vi "Write I16.vi"(6 "wait for reply (T)":bool=TRUE, 7 "Data":i16, 8 "error in":errorcluster, 9 "Variable":string, 10 "Drive":string) -> (0 "error out":errorcluster, 1 "timed out?":bool)   [LabVIEW 2024, in "Hardware Controller.lvlib"]
doc: "This event will pass on the data to be written to the ethercat module\n_____\nCreated using DQMH Event Scripter 7.0.0.1280."
uses:
  Hardware Controller.lvlib
  Write I16 Argument--cluster.ctl
  Write I16 (Reply Payload)--cluster.ctl
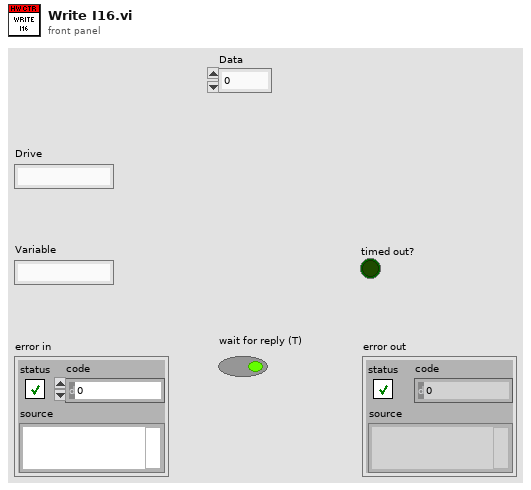
[diagram p1: front panel]
types:
  T1 = typedef "Hardware Controller.lvlib/Write I16 Argument--cluster.ctl" = cluster{"Drive":string, "Variable":string, "Data":i16, "Wait Notifier":refnum<notifier>, "wait for reply":bool}
  T2 = typedef "Hardware Controller.lvlib/Request Events--cluster.ctl" = cluster{"Stop Module":refnum<user-event>, "Show Panel":refnum<user-event>, "Hide Panel":refnum<user-event>, "Get Module Execution Status":refnum<user-event>, "Show Diagram":refnum<user-event>, "Private":cluster{"Start System State Broadcast Helper Loop":refnum<user-event>, "Launch EtherCat":refnum<user-event>}, "Launch all Hardware":refnum<user-event>, "Write I16":refnum<user-event>}
  T3 = typedef "Hardware Controller.lvlib/Write I16 (Reply Payload)--cluster.ctl" = cluster{"error":errorcluster}
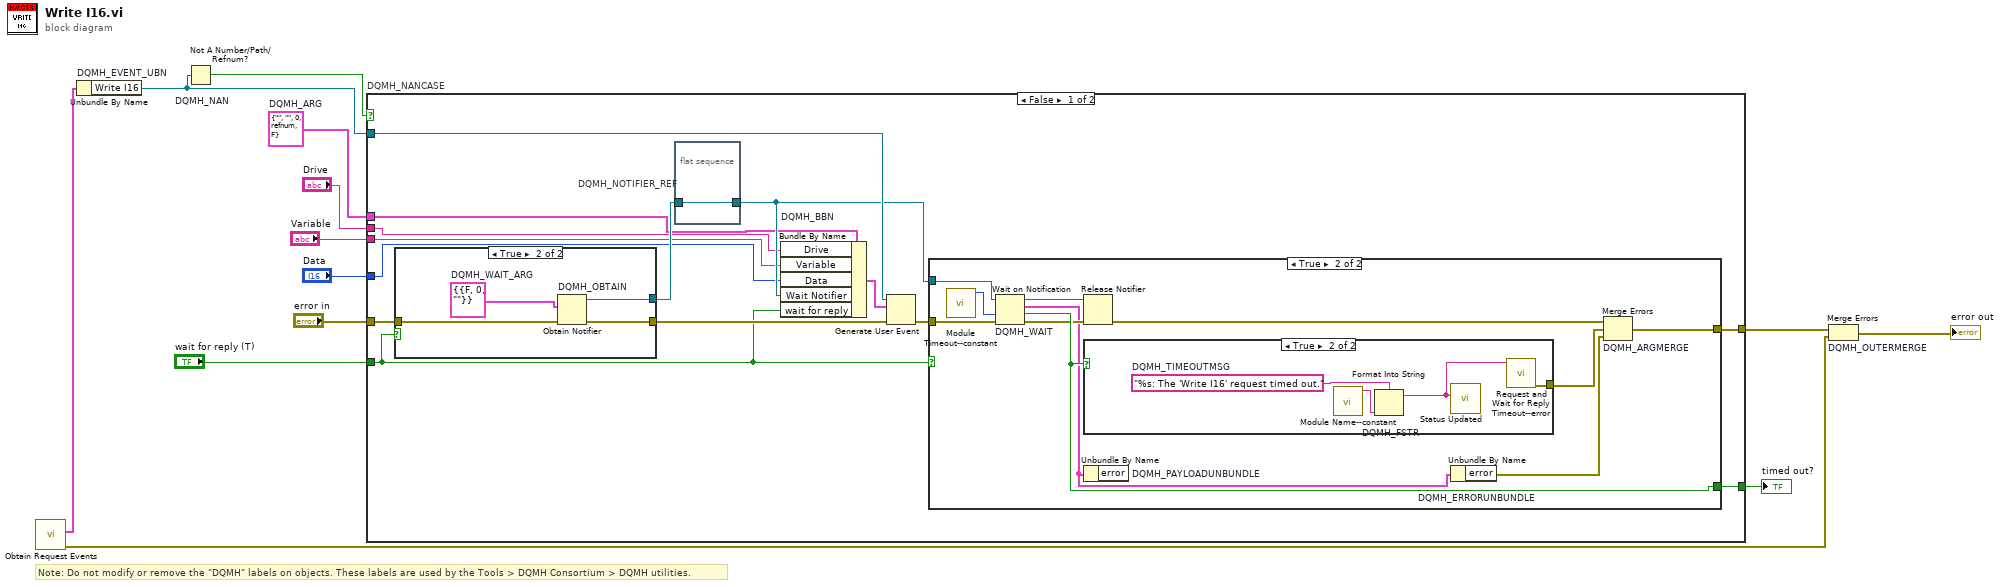
[diagram p0: block diagram]
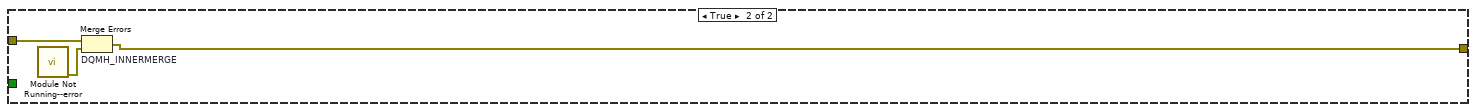
[diagram p5: hidden frame]
diagram:
  w7 = T1 {"Drive"="", "Variable"="", "Data"=0, "Wait Notifier"=refnum, "wait for reply"=FALSE}  # DQMH_ARG
  # "Note: Do not modify or remove the \"DQMH\" labels on objects. These labels are used by the Tools > DQMH Consortium > DQMH utilities."
  n1 = call "Obtain Request Events.vi"() -> ("error out"=w2:errorcluster, "Hardware Controller Request Events"=w1:T2)  [unwired: 10 in]
  n2 = Unbundle By Name "DQMH_EVENT_UBN"(w1) -> ("Write I16"=w11:refnum<user-event>)
  n3 = Not A Number/Path/Refnum? "DQMH_NAN"(number/path/refnum=w11) -> (NaN/Path/Refnum?=w10:bool)
  n4 = case "DQMH_NANCASE" shown="False" w10 {
    tunnel: "error in" -> [w27 w52]
    tunnel: w11 -> [w25 _]
    tunnel: [w22 w51] -> w8
    tunnel: [w23 _] -> w9
    tunnel: w7 -> [w18 _]
    tunnel: "Drive" -> [w17 _]
    tunnel: "Variable" -> [w16 _]
    tunnel: "Data" -> [w15 _]
    tunnel: "wait for reply (T)" -> [w14 _]
    frame False {
      n5 = case shown="True" w14 {
        tunnel: w27 -> [w45 w49]
        tunnel: [w45 w48] -> w24
        tunnel: [_ w46] -> w20
        frame False {
        }
        frame True {
          w47 = T3 {"error"={"status"=FALSE, "code"=0, "source"=""}}  # DQMH_WAIT_ARG
          n6 = Obtain Notifier "DQMH_OBTAIN"(notification data type=w47, error in (no error)=w49) -> (notifier out=w46:refnum<notifier>, error out=w48:errorcluster)  [unwired: 2 in, 1 out]
        }
      }
      n7 = flat-sequence "DQMH_NOTIFIER_REF" {
        tunnel: w20 -> [w28]
        tunnel: [w28] -> w19
        frame #0 {
        }
      }
      n8 = Bundle By Name "DQMH_BBN"(cluster=w18, "Drive"=w17, "Variable"=w16, "Data"=w15, "Wait Notifier"=w19, "wait for reply"=w14) -> (w21:T1)
      n9 = Generate User Event(user event=w25, event data cluster=w21, error in=w24) -> (error out=w26:errorcluster)  [unwired: 1 in, 1 out]
      n10 = case shown="True" w14 {
        tunnel: w26 -> [w29 w40]
        tunnel: w19 -> [_ w39]
        tunnel: [_ w37] -> w23
        tunnel: [w29 w36] -> w22
        frame False {
        }
        frame True {
          n11 = call "Module Timeout--constant.vi"() -> ("Module Timeout"=w30:i32)  [unwired: 11 in]
          n12 = Wait on Notification "DQMH_WAIT"(notifier=w39, timeout in ms (-1)=w30, error in (no error)=w40) -> (notifier out=w38:refnum<notifier>, notification=w31:T3, timed out?=w37:bool, error out=w35:errorcluster)  [unwired: 1 in]
          n13 = Release Notifier(notifier=w38, error in (no error)=w35) -> (error out=w34:errorcluster)  [unwired: 1 in, 2 out]
          n14 = case shown="True" w37 {
            tunnel: [_ w42] -> w32
            frame False {
            }
            frame True {
              w44 = "%s: The 'Write I16' request timed out."  # DQMH_TIMEOUTMSG
              n15 = call "Module Name--constant.vi"() -> ("Module Name"=w41:string)  [unwired: 11 in]
              n16 = Format Into String "DQMH_FSTR"(format string=w44, w41) -> (resulting string=w43:string)  [unwired: 2 in, 1 out]
              n17 = call "Status Updated.vi"("Status"=w43) -> ()  [unwired: 10 in, 1 out]
              n18 = call "Request and Wait for Reply Timeout--error.vi"("Error Message"=w43) -> ("error out"=w42:errorcluster)  [unwired: 10 in]
            }
          }
          n19 = Unbundle By Name "DQMH_PAYLOADUNBUNDLE"(w31) -> ()  [unwired: 1 out]
          n20 = Unbundle By Name "DQMH_ERRORUNBUNDLE"(w31) -> ("error"=w33:errorcluster)
          n21 = Merge Errors "DQMH_ARGMERGE"(w34, w32, w33) -> (w36:errorcluster)
        }
      }
    }
    frame True {
      n22 = call "Module Not Running--error.vi"() -> ("error out"=w50:errorcluster)  [unwired: 11 in]
      n23 = Merge Errors "DQMH_INNERMERGE"(w52, w50) -> (w51:errorcluster)
    }
  }
  "timed out?" <- w9
  n24 = Merge Errors "DQMH_OUTERMERGE"(w8, w2) -> (→"error out":errorcluster)
